vi "Read Altura.vi"(8 "error in (no error)":errorcluster, 11 "Triangulo in":refnum<class "Triangulo.lvclass">) -> (0 "error out":errorcluster, 2 "Altura":dbl, 3 "Triangulo out":refnum<class "Triangulo.lvclass">)   [LabVIEW 2024, in "Triangulo.lvclass"]
uses:
  Triangulo.lvclass
  Triangulo.lvclass/Triangulo.ctl
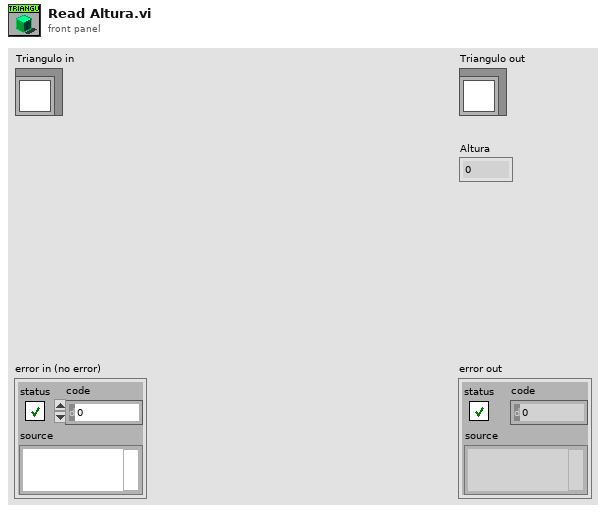
[diagram p1: front panel]
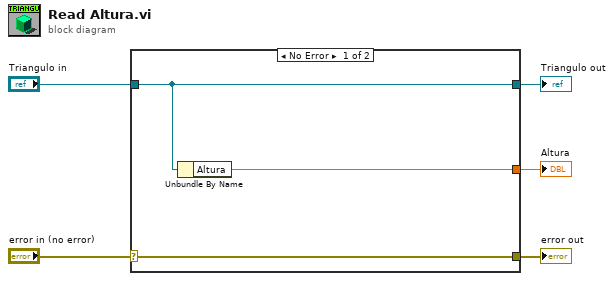
[diagram p0: block diagram]
diagram:
  n1 = case shown="No Error" "error in (no error)" {
    selector: "error in (no error)" -> [w8 w9]
    tunnel: [w8 w9] -> w4
    tunnel: [w7 w10] -> w2
    tunnel: "Triangulo in" -> [w7 w10]
    tunnel: [w6 _] -> w1
    frame No Error {
      n2 = Unbundle By Name(w7) -> ("Altura"=w6:dbl)
    }
    frame Error {
    }
  }
  "error out" <- w4
  "Triangulo out" <- w2
  "Altura" <- w1
